vi "Relay Data.vi"   [LabVIEW 2011]
doc: "This VI relays information to the simulator."
uses:
  Global Variables.vi
panel:
  # "This VI relays information to the AFM simulation."
types:
  T1 = cluster{"Image Height":dbl, "Image Width":dbl, "X Offset":dbl, "Y Offset":dbl}
  T2 = cluster{"Old Image Height":dbl, "Old Image Width":dbl, "Old X Offset":dbl, "Old Y Offset":dbl}
  T3 = cluster{"Old X":dbl, "Old Y":dbl, "Old Voltage":dbl, "Old Wire Width":dbl, "Old Center of Vision":string, "Old Visible":bool, "Old RGB Value":u32}
  T4 = cluster{"X":dbl, "Y":dbl, "Voltage":dbl, "Wire Width":dbl, "Center of Vision":string, "Visible":bool, "RGB Value":u32}
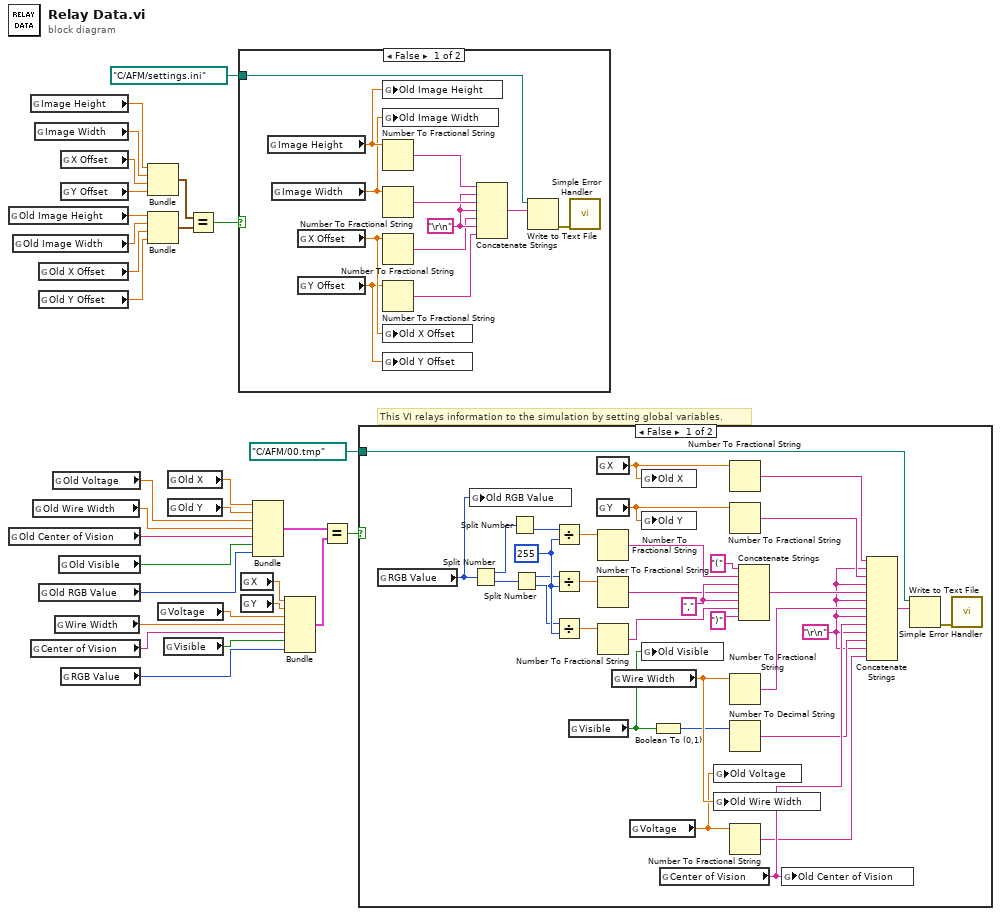
[diagram p0: block diagram]
diagram:
  # "This VI relays information to the simulation by setting global variables."
  n1 = global read "Global Variables.vi" "Old Image Height"() -> (w9:dbl)
  n2 = global read "Global Variables.vi" "Old Center of Vision"() -> (w25:string)
  n3 = global read "Global Variables.vi" "Old Image Width"() -> (w8:dbl)
  n4 = global read "Global Variables.vi" "Image Height"() -> (w13:dbl)
  n5 = global read "Global Variables.vi" "Center of Vision"() -> (w19:string)
  n6 = global read "Global Variables.vi" "Old Wire Width"() -> (w26:dbl)
  n7 = global read "Global Variables.vi" "Image Width"() -> (w12:dbl)
  n8 = global read "Global Variables.vi" "Old X Offset"() -> (w7:dbl)
  n9 = global read "Global Variables.vi" "Old Y Offset"() -> (w6:dbl)
  n10 = global read "Global Variables.vi" "Old RGB Value"() -> (w15:u32)
  n11 = global read "Global Variables.vi" "Old Voltage"() -> (w27:dbl)
  n12 = global read "Global Variables.vi" "Wire Width"() -> (w20:dbl)
  n13 = global read "Global Variables.vi" "Old Visible"() -> (w24:bool)
  n14 = global read "Global Variables.vi" "X Offset"() -> (w11:dbl)
  n15 = global read "Global Variables.vi" "Y Offset"() -> (w10:dbl)
  n16 = global read "Global Variables.vi" "RGB Value"() -> (w14:u32)
  n17 = Bundle("Image Height"=w13, "Image Width"=w12, "X Offset"=w11, "Y Offset"=w10) -> (w5:T1)  [unwired: 1 in]
  n18 = Bundle("Old Image Height"=w9, "Old Image Width"=w8, "Old X Offset"=w7, "Old Y Offset"=w6) -> (w4:T2)  [unwired: 1 in]
  n19 = global read "Global Variables.vi" "Voltage"() -> (w21:dbl)
  n20 = global read "Global Variables.vi" "Visible"() -> (w18:bool)
  n21 = global read "Global Variables.vi" "Old X"() -> (w29:dbl)
  n22 = global read "Global Variables.vi" "Old Y"() -> (w28:dbl)
  n23 = Equal?(x=w5, y=w4) -> (x = y?=w3:bool)
  n24 = case shown="False" w3 {
    tunnel: path "C:/AFM/settings.ini" ("base path") -> [w38 _]
    frame False {
      w35 = "\r\n"
      n25 = global read "Global Variables.vi" "Image Height"() -> (w37:dbl)
      n26 = global read "Global Variables.vi" "Image Width"() -> (w36:dbl)
      n27 = global read "Global Variables.vi" "X Offset"() -> (w34:dbl)
      n28 = global read "Global Variables.vi" "Y Offset"() -> (w33:dbl)
      n29 = global write "Global Variables.vi" "Old Image Height"(w37) -> ()
      n30 = global write "Global Variables.vi" "Old Image Width"(w36) -> ()
      n31 = Number To Fractional String(number=w37) -> (F-format string=w42:string)  [unwired: 3 in]
      n32 = Number To Fractional String(number=w36) -> (F-format string=w41:string)  [unwired: 3 in]
      n33 = Number To Fractional String(number=w34) -> (F-format string=w32:string)  [unwired: 3 in]
      n34 = Number To Fractional String(number=w33) -> (F-format string=w31:string)  [unwired: 3 in]
      n35 = global write "Global Variables.vi" "Old X Offset"(w34) -> ()
      n36 = global write "Global Variables.vi" "Old Y Offset"(w33) -> ()
      n37 = Concatenate Strings(w42, w35, w41, w35, w32, w35, w31) -> (w40:string)
      n38 = Write to Text File(file (use dialog)=w38, text=w40) -> (error out=w39:errorcluster)  [unwired: 2 in, 2 out]
      n39 = call <vilib>:"Simple Error Handler.vi"("error in (no error)"=w39) -> ()  [unwired: 4 in, 5 out]
    }
    frame True {
    }
  }
  n40 = global read "Global Variables.vi" "X"() -> (w23:dbl)
  n41 = global read "Global Variables.vi" "Y"() -> (w22:dbl)
  n42 = Bundle("Old X"=w29, "Old Y"=w28, "Old Voltage"=w27, "Old Wire Width"=w26, "Old Center of Vision"=w25, "Old Visible"=w24, "Old RGB Value"=w15) -> (w17:T3)  [unwired: 1 in]
  n43 = Bundle("X"=w23, "Y"=w22, "Voltage"=w21, "Wire Width"=w20, "Center of Vision"=w19, "Visible"=w18, "RGB Value"=w14) -> (w16:T4)  [unwired: 1 in]
  n44 = Equal?(x=w17, y=w16) -> (x = y?=w30:bool)
  n45 = case shown="False" w30 {
    tunnel: path "C:/AFM/00.tmp" ("file (use dialog)") -> [w71 _]
    frame False {
      w54 = u8 255 ("y")
      w59 = "," ("string")
      w51 = "\r\n"
      n46 = global read "Global Variables.vi" "RGB Value"() -> (w43:u32)
      n47 = global write "Global Variables.vi" "Old RGB Value"(w43) -> ()
      n48 = Split Number(x=w43) -> (hi(x)=w48:u16, lo(x)=w49:u16)
      n49 = Split Number(x=w48) -> (lo(x)=w46:u8)  [unwired: 1 out]
      n50 = Split Number(x=w49) -> (hi(x)=w45:u8, lo(x)=w44:u8)
      n51 = Divide(x=w46, y=w54) -> (x/y=w55:dbl)
      n52 = Divide(x=w45, y=w54) -> (x/y=w52:dbl)
      n53 = Divide(x=w44, y=w54) -> (x/y=w53:dbl)
      n54 = global read "Global Variables.vi" "Visible"() -> (w65:bool)
      n55 = global read "Global Variables.vi" "X"() -> (w70:dbl)
      n56 = global read "Global Variables.vi" "Y"() -> (w69:dbl)
      n57 = Number To Fractional String(number=w55) -> (F-format string=w60:string)  [unwired: 3 in]
      n58 = Number To Fractional String(number=w52) -> (F-format string=w58:string)  [unwired: 3 in]
      n59 = Number To Fractional String(number=w53) -> (F-format string=w57:string)  [unwired: 3 in]
      n60 = global read "Global Variables.vi" "Wire Width"() -> (w68:dbl)
      n61 = global read "Global Variables.vi" "Voltage"() -> (w47:dbl)
      n62 = global write "Global Variables.vi" "Old X"(w70) -> ()
      n63 = global write "Global Variables.vi" "Old Y"(w69) -> ()
      n64 = global write "Global Variables.vi" "Old Visible"(w65) -> ()
      n65 = Boolean To (0,1)(Boolean=w65) -> (0, 1=w64:i16)
      n66 = global read "Global Variables.vi" "Center of Vision"() -> (w67:string)
      n67 = global write "Global Variables.vi" "Old Voltage"(w47) -> ()
      n68 = global write "Global Variables.vi" "Old Wire Width"(w68) -> ()
      n69 = Number To Fractional String(number=w70) -> (F-format string=w75:string)  [unwired: 3 in]
      n70 = Number To Fractional String(number=w69) -> (F-format string=w74:string)  [unwired: 3 in]
      n71 = Number To Fractional String(number=w68) -> (F-format string=w66:string)  [unwired: 3 in]
      n72 = Number To Decimal String(number=w64) -> (decimal integer string=w63:string)  [unwired: 1 in]
      n73 = Number To Fractional String(number=w47) -> (F-format string=w50:string)  [unwired: 3 in]
      n74 = Concatenate Strings("(" ("string"), w60, w59, w58, w59, w57, ")" ("string")) -> (w62:string)
      n75 = global write "Global Variables.vi" "Old Center of Vision"(w67) -> ()
      n76 = Concatenate Strings(w75, w51, w74, w51, w62, w51, w66, w51, w67, w51, w63, w51, w50) -> (w73:string)
      n77 = Write to Text File(file (use dialog)=w71, text=w73) -> (error out=w72:errorcluster)  [unwired: 2 in, 2 out]
      n78 = call <vilib>:"Simple Error Handler.vi"("error in (no error)"=w72) -> ()  [unwired: 4 in, 5 out]
    }
    frame True {
    }
  }
